vi "WaitForFRPQuery.vi"(0 "System no.":i32=1, 1 "Routines to query":string[](array[string]), 3 "Query all routines?":bool, 4 "Option":i32[](array[numeric]), 5 "error in":errorcluster, 7 "Timeout / ms":u32=60000, 8 "Stop refnum":refnum<vi>) -> (19 "error out":errorcluster)   [LabVIEW 2020]
doc: "This vi queries FRP? until the desired option or the timeout has been reached.\nIf the Stop button is pressed, #24 will be sent to the controller and all motion including fast routine scan procedures will be stopped.\n\nValid for C-887, E-712\n\nC-887, E-712: Check HLP? answer to find out if FRP? is supported."
panel:
  in  "Polling time in ms":u32=1
  in  "Stop":bool
  # "This VI queries FRP? until the desired status or timeout has been reached."
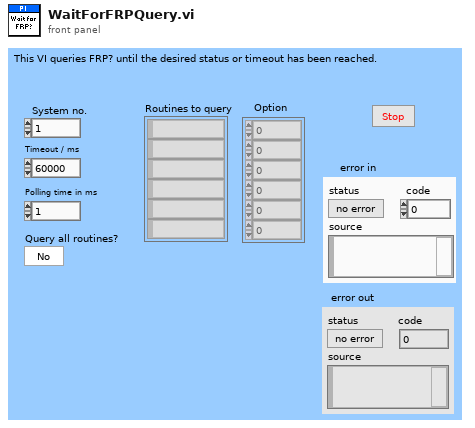
[diagram p1: front panel]
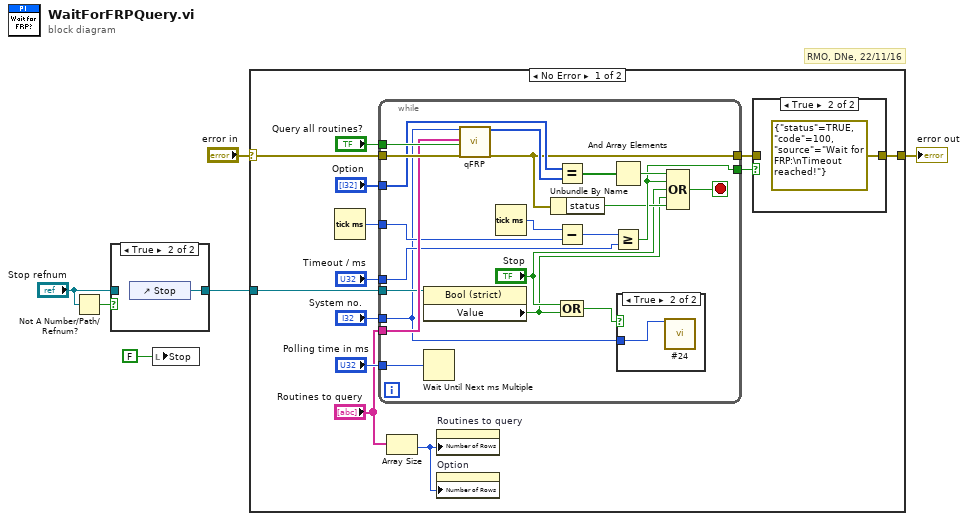
[diagram p0: block diagram]
diagram:
  # "RMO, DNe, 22/11/16"
  n1 = Not A Number/Path/Refnum?(number/path/refnum="Stop refnum") -> (NaN/Path/Refnum?=w4:bool)
  n2 = case shown="True" w4 {
    tunnel: [w7 w8] -> w1
    tunnel: "Stop refnum" -> [w7 _]
    frame False {
    }
    frame True {
      n3 = control-ref of="Stop"() -> (w8:refnum<vi>)
    }
  }
  n4 = local write "Stop"(FALSE ("Local stop")) -> ()
  n5 = case shown="No Error" "error in" {
    selector: "error in" -> [w14 w46]
    tunnel: [w16 w46] -> w5
    tunnel: w1 -> [w12 _]
    frame No Error {
      n6 = Tick Count (ms)() -> (millisecond timer value=w19:u32)
      n7 = while {
        tunnel: w14 -> [w44]
        tunnel: [w30] -> w17
        tunnel: "System no." -> [w24]
        tunnel: "Query all routines?" -> [w43]
        tunnel: "Routines to query" -> [w42]
        tunnel: w19 -> [w40]
        tunnel: "Timeout / ms" -> [w38]
        tunnel: [w31] -> w15
        tunnel: "Option" -> [w36]
        tunnel: w12 -> [w34]
        tunnel: "Polling time in ms" -> [w25]
        stop <- w33 stop-if-true
        n8 = property class="Bool (strict)"(reference=w34) -> ("Value"=w26:bool)  [unwired: 1 in, 2 out]
        n9 = Wait Until Next ms Multiple(millisecond multiple=w25) -> ()  [unwired: 1 out]
        n10 = call "qFRP.vi"("System no."=w24, "Routines to query"=w42, "All routines?"=w43, "error in"=w44) -> ("Status"=w37:i32[], "error out"=w30:errorcluster)  [unwired: 14 out]
        n11 = Tick Count (ms)() -> (millisecond timer value=w41:u32)
        n12 = Unbundle By Name(w30) -> ("status"=w29:bool)
        n13 = Equal?(x=w36, y=w37) -> (x = y?=w35:bool[])
        n14 = Subtract(x=w41, y=w40) -> (x-y=w39:u32)
        n15 = Compound Arithmetic op=OR("Stop", w26) -> (w28:bool)
        n16 = And Array Elements(Boolean array=w35) -> (logical AND=w32:bool)
        n17 = Greater Or Equal?(x=w39, y=w38) -> (x >= y?=w31:bool)
        n18 = case shown="True" w28 {
          tunnel: w24 -> [_ w45]
          frame False {
          }
          frame True {
            n19 = call "#24.vi"("System no."=w45) -> ()  [unwired: 1 in, 18 out]
          }
        }
        n20 = Compound Arithmetic op=OR(w32, w31, "Stop", w26, w29) -> (w33:bool)
      }
      n21 = Array Size(array="Routines to query") -> (size(s)=w9:i32)
      n22 = property on="Routines to query" class="Arr (strict)"("Number of Rows"=w9) -> ()  [unwired: 2 in, 2 out]
      n23 = property on="Option" class="Arr (strict)"("Number of Rows"=w9) -> ()  [unwired: 2 in, 2 out]
      n24 = case shown="True" w15 {
        tunnel: w17 -> [w22 _]
        tunnel: [w22 errorcluster {"status"=TRUE, "code"=100, "source"="Wait for FRP:\nTimeout reached!"} ("error out")] -> w16
        frame False {
        }
        frame True {
        }
      }
    }
    frame Error {
    }
  }
  "error out" <- w5
